vi "Register.vi"(7 "Event":refnum<class "Event.lvclass">, 8 "Error In":errorcluster, 9 "View Event Fire Handler":refnum<class "Abstract Event Message for View.lvclass">, 10 "Registrant Details":T1, 11 "Controller Actor In":refnum<class "Controller Actor.lvclass">) -> (0 "Error Out":errorcluster, 3 "Controller Actor Out":refnum<class "Controller Actor.lvclass">)   [LabVIEW 2016, in "Event Actors.lvlib" / "Controller Actor.lvclass"]
doc: "This method registers a specific Actors Enqueuer and a Zero Coupling based message (inheriting from Event Generated Msg.lvclass) to used when the specified Event is Fired anywhere inside the Event Source Actor."
uses:
  Controller Actor.lvclass
  Event/Event.lvclass
  View Details.ctl
  <vilib>/ActorFramework/Message Enqueuer/Message Enqueuer.lvclass
  Event Handlers/Abstract Event Message for View/Abstract Event Message for View.lvclass
  Controller Actor.lvclass/Controller Actor.ctl
  Event Handler Details.ctl
  Event/Event.lvclass/Event.ctl
  <vilib>/Utility/error.llb/Error Cluster From Error Code.vi
  <vilib>/ErrorRing/Error Ring.xnode
  <resource>/AFDebug/AF Debug.lvlib
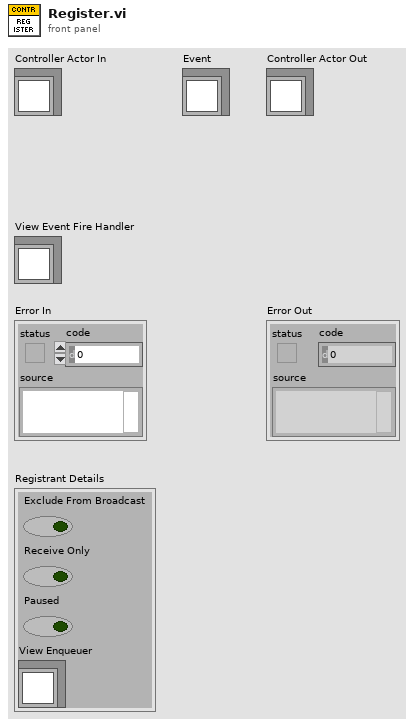
[diagram p1: front panel]
types:
  T1 = typedef "Event Actors.lvlib/Controller Actor.lvclass/View Details.ctl" = cluster{"Exclude From Broadcast":bool, "Receive Only":bool, "Paused":bool, "View Enqueuer":refnum<class "Message Enqueuer.lvclass">}
  T2 = typedef "Event Actors.lvlib/Controller Actor.lvclass/Event Handler Details.ctl" = cluster{"Exclude From Broadcast":bool, "Paused":bool, "View Event Fire Handler":refnum<class "Abstract Event Message for View.lvclass">}
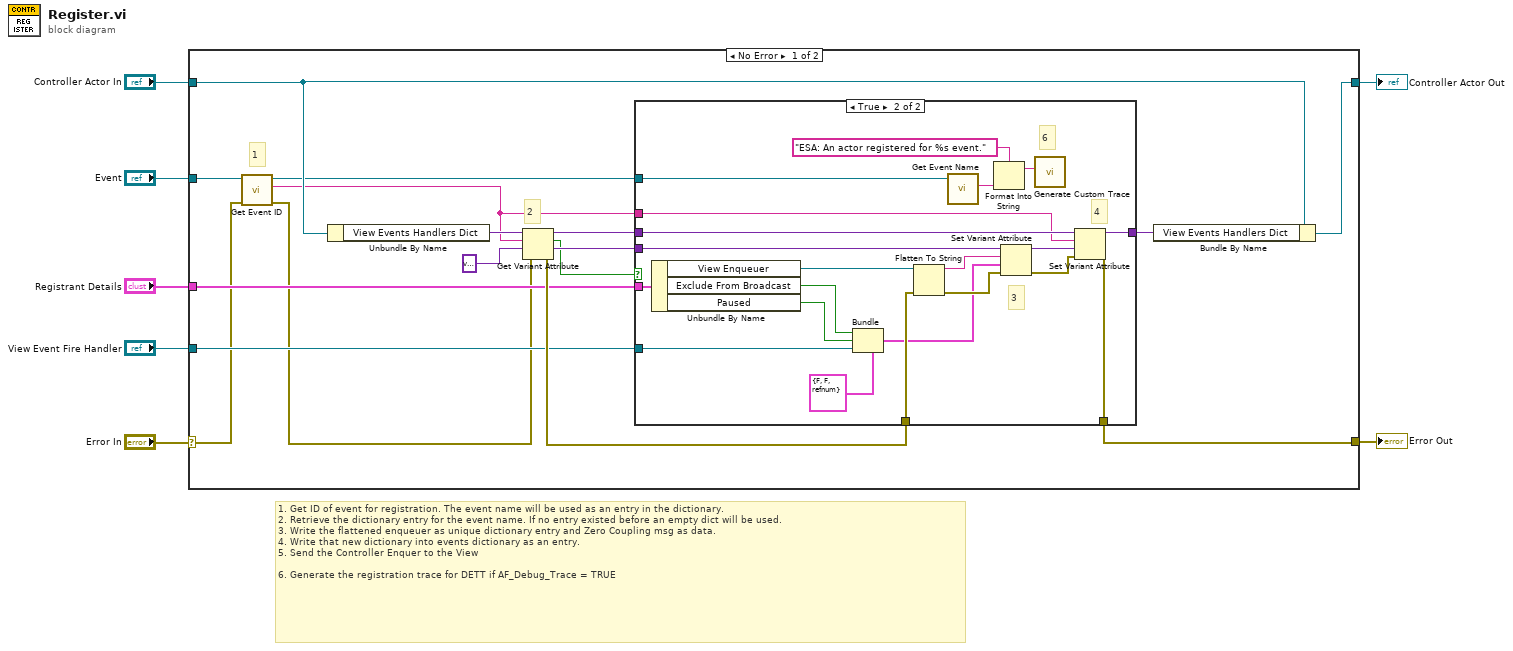
[diagram p0: block diagram]
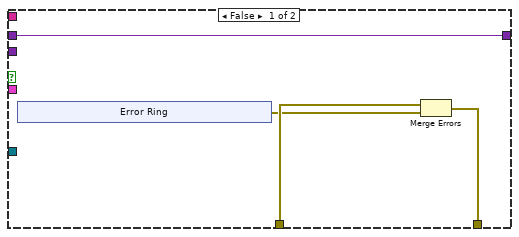
[diagram p2: hidden frame]
diagram:
  # "1. Get ID of event for registration. The event name will be used as an entry in the dictionary.\n2. Retrieve the dictionary entry for the event name. If no entry existed before an empty dict will be used.\n3. Write the flattened enqueuer as unique dictionary entry and Zero Coupling msg as data.\n4. Write that new dictionary into events dictionary as an entry.\n5. Send the Controller Enquer to the View\n\n6. Generate the registration trace for DETT if AF_Debug_Trace = TRUE"
  n1 = case shown="No Error" "Error In" {
    selector: "Error In" -> [w12 w54]
    tunnel: "Controller Actor In" -> [w14 w55]
    tunnel: "Event" -> [w13 _]
    tunnel: [w20 w55] -> w6
    tunnel: [w24 w54] -> w4
    tunnel: "Registrant Details" -> [w15 _]
    tunnel: "View Event Fire Handler" -> [w19 _]
    frame No Error {
      # "2"
      # "1"
      n2 = call-dynamic "Get Event ID.vi"("error in (no error)"=w12, "Event in"=w13) -> ("error out"=w10:errorcluster, "Event ID"=w11:string, "Event out"=w8:refnum<class "Event.lvclass">)  [unwired: 7 in]
      n3 = Unbundle By Name(w14) -> ("View Events Handlers Dict"=w23:variant)
      n4 = Get Variant Attribute(Variant=w23, name=w11, default value (empty Variant)=variant ("variant"), error in=w10) -> (duplicate Variant=w22:variant, found=w9:bool, value=w17:variant, error out=w21:errorcluster)
      n5 = case shown="True" w9 {
        tunnel: [w27 w53] -> w24
        tunnel: w22 -> [w26 w52]
        tunnel: w21 -> [w28 w51]
        tunnel: w19 -> [_ w34]
        tunnel: [w26 w48] -> w18
        tunnel: w17 -> [_ w47]
        tunnel: w15 -> [_ w39]
        tunnel: w11 -> [_ w46]
        tunnel: w8 -> [_ w40]
        frame False {
          n6 = xnode "Error Ring"() -> ("error out"=w25:errorcluster)
          n7 = Merge Errors(w28, w25) -> (w27:errorcluster)
        }
        frame True {
          # "6"
          # "4"
          # "3"
          n8 = Unbundle By Name(w39) -> ("View Enqueuer"=w38:refnum<class "Message Enqueuer.lvclass">, "Exclude From Broadcast"=w36:bool, "Paused"=w35:bool)
          n9 = Bundle(cluster=T2 {"Exclude From Broadcast"=FALSE, "Paused"=FALSE, "View Event Fire Handler"=refnum} ("Sink Settings"), "Exclude From Broadcast"=w36, "Paused"=w35, "View Event Fire Handler"=w34) -> (w33:T2)
          n10 = Flatten To String(anything=w38, error in (no error)=w51) -> (data string=w50:string, error out=w45:errorcluster)  [unwired: 2 in, 1 out]
          n11 = call "Get Event Name.vi"("Event In"=w40) -> ("Name"=w41:string)  [unwired: 9 in, 1 out]
          n12 = Format Into String(format string="ESA: An actor registered for %s event." ("Custom Action"), w41) -> (resulting string=w42:string)  [unwired: 2 in, 1 out]
          n13 = Set Variant Attribute(Variant=w47, name=w50, value=w33, error in=w45) -> (Variant out=w49:variant, error out=w44:errorcluster)  [unwired: 1 out]
          n14 = call <resource>:"Generate Custom Trace.vi"("Custom Action"=w42) -> ()  [unwired: 11 in]
          n15 = Set Variant Attribute(Variant=w52, name=w46, value=w49, error in=w44) -> (Variant out=w48:variant, error out=w53:errorcluster)  [unwired: 1 out]
        }
      }
      n16 = Bundle By Name(cluster=w14, "View Events Handlers Dict"=w18) -> (w20:refnum<class "Controller Actor.lvclass">)
    }
    frame Error {
    }
  }
  "Error Out" <- w4
  "Controller Actor Out" <- w6
